vi "Get Form Names.vi"(8 "error in (no error)":errorcluster, 11 "Request in":refnum<class "Request.lvclass">) -> (0 "error out":errorcluster, 2 "Form Names":string[](array[string]), 3 "Request out":refnum<class "Request.lvclass">)   [LabVIEW 2020, in "HTTP Utils.lvlib" / "Request.lvclass"]
uses:
  Request.lvclass
  Request.lvclass/Request.ctl
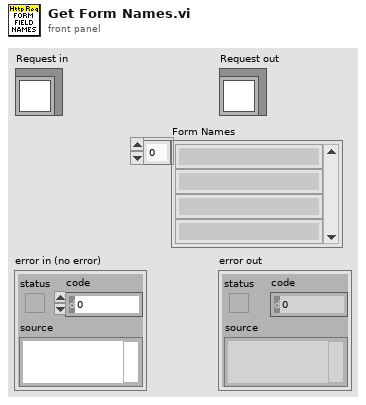
[diagram p1: front panel]
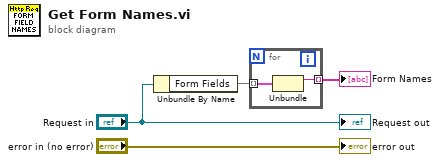
[diagram p0: block diagram]
diagram:
  n1 = Unbundle By Name("Request in") -> ("Form Fields"=w2:map{string, refnum<class "FormField.lvclass">})
  n2 = for {
    tunnel: w2 -> [w6] mode=indexing
    tunnel: [w5] -> w1 mode=indexing
    n3 = Unbundle(w6) -> (w5:string)  [unwired: 1 out]
  }
  "Form Names" <- w1
  "error out" <- "error in (no error)"
  "Request out" <- "Request in"
